vi "UART Write.vi"(8 "Error In":errorcluster, 9 "Data":u8[](array[numeric]), 10 "UART Channel":u8, 11 "LINX Device Config":T1) -> (0 "Error Out":errorcluster, 3 "LINX Device Config":T1)   [LabVIEW 2011, in "LVH-LINX.lvlib" / "Device.lvlib"]
doc: "Transmit data using the specified UART channel."
uses:
  Device.lvlib
  Type Defs/LINX Device Config.ctl
  Type Defs/Interface.ctl
  Type Defs/TCP Config.ctl
  Type Defs/Device Family.ctl
  Type Defs/Error Type.ctl
  LVH-LINX.lvlib
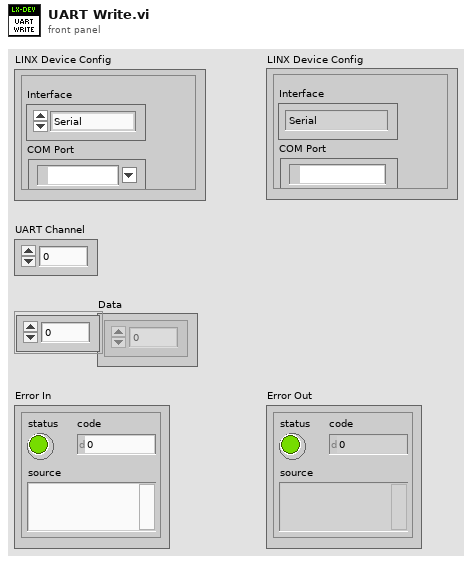
[diagram p1: front panel]
types:
  T1 = typedef "LVH-LINX.lvlib/Device.lvlib/LINX Device Config.ctl" = cluster{"Interface":T2, "COM Port":refnum<visa-resource-name>, "TCP Configuration":T3, "Device Family":T4, "Device ID":u8, "Device Name":string, "TCP Ref":refnum<k5>}
  T2 = typedef "LVH-LINX.lvlib/Interface.ctl" = enum16{"Serial", "TCP"}
  T3 = typedef "LVH-LINX.lvlib/Device.lvlib/TCP Config.ctl" = cluster{"IP Address":string, "Port":u16}
  T4 = typedef "LVH-LINX.lvlib/Device Family.ctl" = enum8{"National Instruments", "Digilent", "Arduino"}
  T5 = typedef "LVH-LINX.lvlib/Error Type.ctl" = enum16{"Unknown", "Timeout", "Corrupt Return Packet", "Unable To Connect", "Command Not Supported", "Channel DNE"}
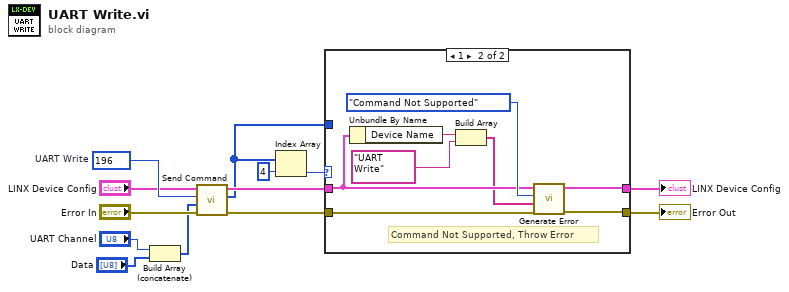
[diagram p0: block diagram]
diagram:
  w12 = u16 196  # UART Write
  n1 = Build Array (concatenate)("UART Channel", "Data") -> (w3:u8[])
  n2 = call "Send Command.vi"("Error In"="Error In", "ARGS"=w3, "CMD"=w12, "LINX Device Config"="LINX Device Config") -> ("Error Out"=w5:errorcluster, "Response"=w2:u8[], "LINX Device Config"=w7:T1)  [unwired: 5 in]
  n3 = Index Array(array=w2, index=4) -> (element=w9:u8)
  n4 = case shown="1" w9 {
    tunnel: [w15 w21] -> w8
    tunnel: w7 -> [w15 w17]
    tunnel: [w14 w22] -> w6
    tunnel: w5 -> [w14 w23]
    tunnel: w2 -> [_ _]
    frame 0, Default {
      # "Status OK, Process Data"
    }
    frame 1 {
      # "Command Not Supported, Throw Error"
      n5 = Unbundle By Name(w17) -> ("Device Name"=w19:string)
      n6 = Build Array(w19, "UART Write") -> (w16:string[])
      n7 = call "Generate Error.vi"("Error In"=w23, "Arguments"=w16, "Error Type"=Error_Type."Command Not Supported", "LINX Device Config"=w17) -> ("Error Out"=w22:errorcluster, "LINX Device Config"=w21:T1)  [unwired: 6 in]
    }
  }
  "Error Out" <- w6
  "LINX Device Config" <- w8
